vi "Force control.vi"() -> ()   [LabVIEW 2021]
uses:
  <vilib>/Platform/TimedLoop/XDataNode/timing_clust.ctl
  <vilib>/Platform/TimedLoop/XDataNode/nitl_modes.ctl
  <vilib>/Platform/TimedLoop/XDataNode/wakeup.ctl
  <vilib>/DAQmx/write.llb/DAQmx Write (Digital Bool 1Line 1Point).vi
  <vilib>/DAQmx/write.llb/DAQmx Write (Analog DBL 1Chan 1Samp).vi
  <vilib>/DAQmx/create/channels.llb/DAQmx Create Channel (AI-Voltage-Basic).vi
  <vilib>/DAQmx/create/channels.llb/DAQmx Create Channel (DO-Digital Output).vi
  <vilib>/DAQmx/create/channels.llb/DAQmx Create Channel (AO-Voltage-Basic).vi
  <vilib>/DAQmx/miscellaneous.llb/DAQmx Fill In Error Info.vi
  <vilib>/addons/control/pid/pid.llb/PID (DBL).vi
  <vilib>/Platform/TimedLoop/XDataNode/XDataNode.xnode
  <vilib>/Platform/TimedLoop/XDataNode/XDNodeRunTimeDep.lvlib
  <vilib>/addons/control/pid/NI_PID_pid.lvlib
panel:
  out "ff_gain 2":dbl
  in  "ff_gain":dbl(slide) scale=0.0..3.0
  out "predict":dbl
  out "Waveform Chart":cluster{"Filtered x":dbl, "Ref Force":dbl}(graph) caption="A"
  out "Total(V)":dbl
  in  "PID ON/OFF":bool
  in  "PID gains":T1={"proportional gain (Kc)"=0.3, "integral time (Ti, min)"=0.1, "derivative time (Td, min)"=0.0} {"derivative time (Td, min)" format="%.3f"; "integral time (Ti, min)" format="%.3f"; "proportional gain (Kc)" format="%.3f"}
  in  "Ref Force":dbl(slide) scale=0.0..40.0
  in  "Motor Enable":bool
  in  "stop":bool
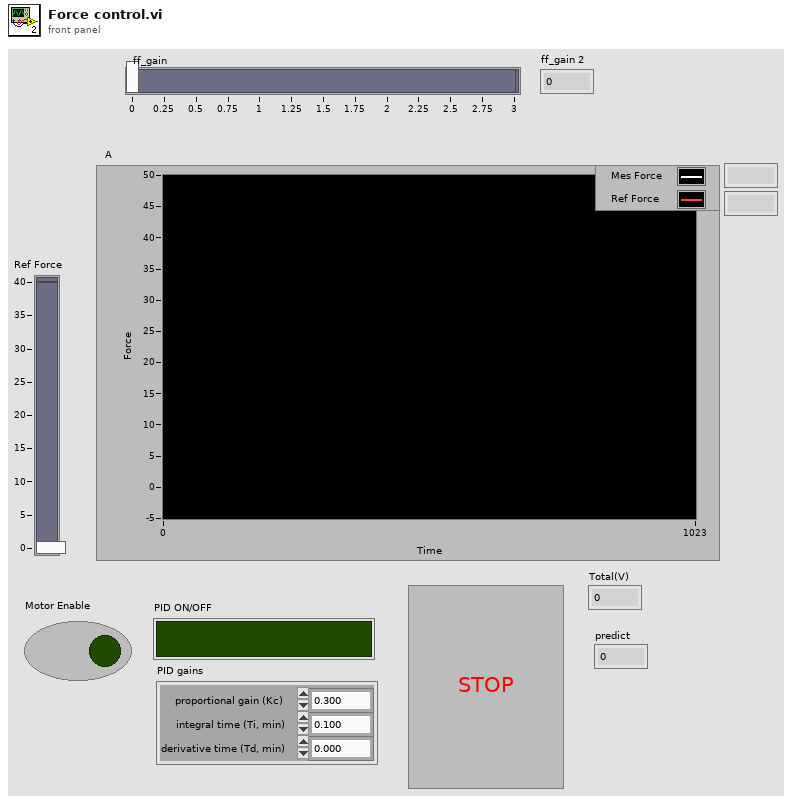
[diagram p1: front panel]
types:
  T1 = cluster{"proportional gain (Kc)":dbl, "integral time (Ti, min)":dbl, "derivative time (Td, min)":dbl}
  T2 = typedef "XDNodeRunTimeDep.lvlib/timing_clust.ctl" = cluster{"Expected End [f-1]":u64, "Actual End [f-1]":u64, "Finished Late? [f-1]":bool, "Expected End [i-1]":u64, "Actual End [i-1]":u64, "Finished Late? [i-1]":bool, "Expected Start [i]":u64, "Actual Start [i]":u64, "Expected Start [f]":u64, "Actual Start [f]":u64, "Source Name":string, "Structure Name":string, "Period":i64, "Deadline":i64, "Offset":i64, "Start":i64, "Priority":i32, "Timeout":i32, "Mode":T3, "Wakeup Reason":T4, "Error":errorcluster, "Source Type":string, "Secondary Source Type":string, "Global End Time":u64, "Global Start Time":u64, "Frame Duration":u64, "Iteration Duration":u64, "Assigned CPU":i32, "I/O Scan Engine Mode":u32}
  T3 = typedef "XDNodeRunTimeDep.lvlib/nitl_modes.ctl" = enum32{"No Change", "Process missed periods, maintain original phase", "Discard missed periods, maintain original phase", "Process missed periods, ignore original phase", "Discard missed periods, ignore original phase"}
  T4 = typedef "XDNodeRunTimeDep.lvlib/wakeup.ctl" = enum32{"Normal", "Aborted", "Asynchronous wakeup", "Timing source error", "Timed loop error", "Timeout"}
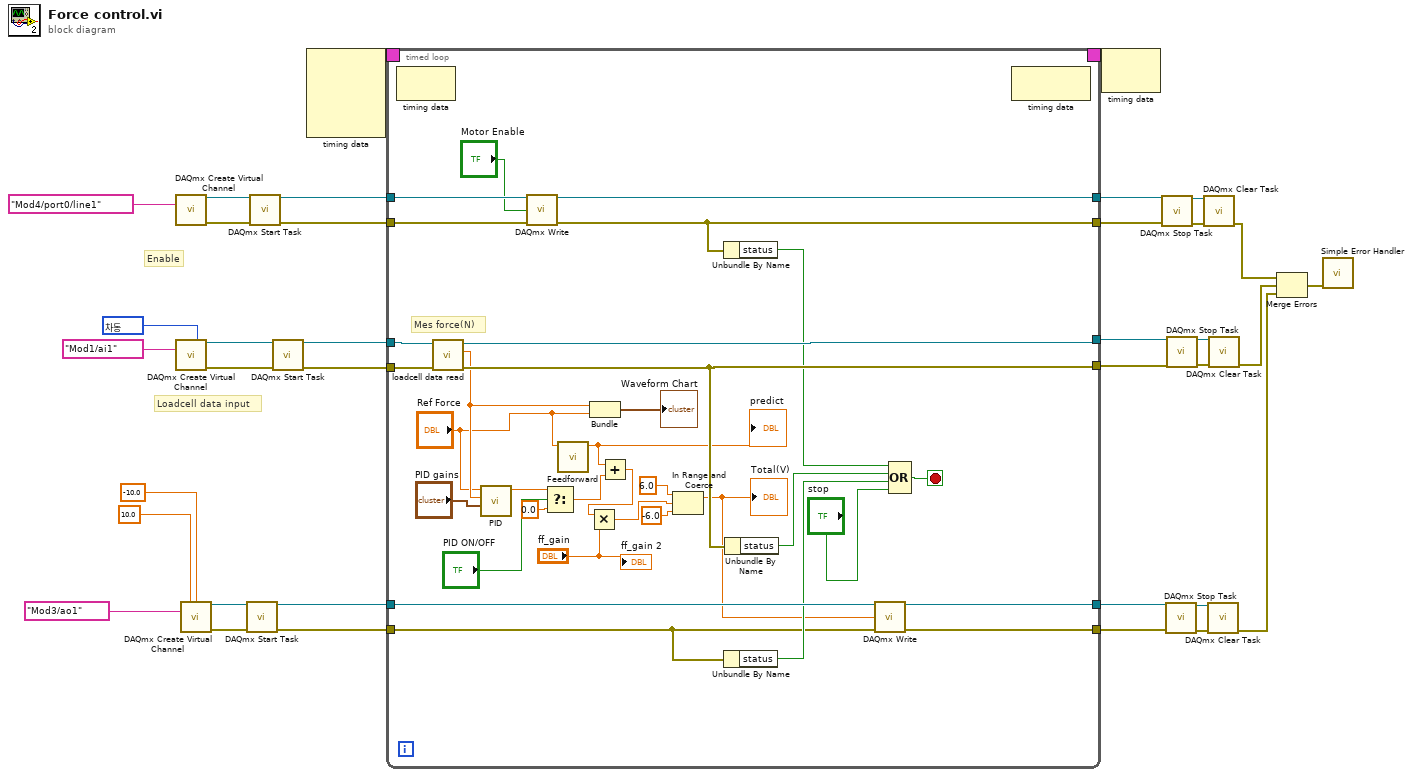
[diagram p0: block diagram]
diagram:
  w25 = 10106 items=["기본"=-1, "RSE"=10083, "NRSE"=10078, "차동"=10106, "유사 차동"=12529] ("input terminal configuration")
  # "Enable"
  # "Loadcell data input"
  n1 = call-poly <vilib>:"DAQmx Create Virtual Channel.vi"("lines"=tag "Mod4/port0/line1") -> ("task out"=w24:refnum<k21>, "error out"=w23:errorcluster)  [unwired: 13 in]
  n2 = call-poly <vilib>:"DAQmx Create Virtual Channel.vi"("input terminal configuration"=w25, "physical channels"=tag "Mod1/ai1") -> ("task out"=w33:refnum<k21>, "error out"=w32:errorcluster)  [unwired: 12 in]
  n3 = call-poly <vilib>:"DAQmx Create Virtual Channel.vi"("maximum value"=10.0, "minimum value"=-10.0, "physical channels"=tag "Mod3/ao1") -> ("task out"=w12:refnum<k21>, "error out"=w11:errorcluster)  [unwired: 11 in]
  n4 = call <vilib>:"DAQmx Start Task.vi"("task/channels in"=w12, "error in"=w11) -> ("task out"=w7:refnum<k21>, "error out"=w6:errorcluster)  [unwired: 12 in]
  n5 = call <vilib>:"DAQmx Start Task.vi"("task/channels in"=w24, "error in"=w23) -> ("task out"=w21:refnum<k21>, "error out"=w20:errorcluster)  [unwired: 12 in]
  n6 = call <vilib>:"DAQmx Start Task.vi"("task/channels in"=w33, "error in"=w32) -> ("task out"=w31:refnum<k21>, "error out"=w30:errorcluster)  [unwired: 12 in]
  n7 = node-c288() -> (w36:T2)  [unwired: 4 in]
  n8 = timed-loop {
    timing: w36 -> [_]
    timing-out: [_] -> w35
    tunnel: w31 -> [w69]
    tunnel: w30 -> [w68]
    tunnel: [w67] -> w26
    tunnel: [w66] -> w27
    tunnel: w21 -> [w63]
    tunnel: w20 -> [w62]
    tunnel: [w60] -> w17
    tunnel: [w59] -> w16
    tunnel: w7 -> [w57]
    tunnel: w6 -> [w52]
    tunnel: [w56] -> w3
    tunnel: [w55] -> w2
    stop <- w64 stop-if-true
    # "Mes force(N)"
    n9 = node-c288() -> ()  [unwired: 1 in, 1 out]
    n10 = call "loadcell data read.vi"("error in (no error)"=w68, "Refnum in"=w69) -> ("error out"=w66:errorcluster, "Filtered x"=w44:dbl, "Refnum out"=w67:refnum<k21>)  [unwired: 7 in]
    n11 = call-poly <vilib>:"PID.vi"("PID gains"="PID gains", "process variable"=w44, "setpoint"="Ref Force") -> ("output"=w50:dbl)  [unwired: 7 in, 1 out]
    n12 = call-poly <vilib>:"DAQmx Write.vi"("task/channels in"=w63, "data"="Motor Enable", "error in"=w62) -> ("task out"=w60:refnum<k21>, "error out"=w59:errorcluster)  [unwired: 10 in, 1 out]
    n13 = Select(t=w50, s="PID ON/OFF", f=0.0) -> (s? t:f=w40:dbl)
    n14 = call "Feedforward.vi"("Ref force"="Ref Force") -> ("predict"=w41:dbl)  [unwired: 10 in]
    "predict" <- w41
    n15 = Bundle("Filtered x"=w44, "Ref Force"="Ref Force") -> (→"Waveform Chart":cluster{"Filtered x":dbl, "Ref Force":dbl})  [unwired: 1 in]
    n16 = Add(x=w41, y=w40) -> (x+y=w39:dbl)
    n17 = Multiply(x=w39, y="ff_gain") -> (x*y=w38:dbl)
    n18 = In Range and Coerce(upper limit=6.0, x=w38, lower limit=-6.0) -> (coerced(x)=w45:dbl)  [unwired: 1 out]
    "Total(V)" <- w45
    n19 = Unbundle By Name(w59) -> ("status"=w58:bool)
    n20 = Unbundle By Name(w52) -> ("status"=w54:bool)
    n21 = Unbundle By Name(w66) -> ("status"=w65:bool)
    n22 = call-poly <vilib>:"DAQmx Write.vi"("task/channels in"=w57, "data"=w45, "error in"=w52) -> ("task out"=w56:refnum<k21>, "error out"=w55:errorcluster)  [unwired: 10 in, 1 out]
    n23 = Compound Arithmetic op=OR(w58, w65, w54, "stop") -> (w64:bool)
    n24 = node-c288() -> ()  [unwired: 1 in, 1 out]
    "ff_gain 2" <- "ff_gain"
  }
  n25 = node-c288(w35) -> ()  [unwired: 1 out]
  n26 = call <vilib>:"DAQmx Stop Task.vi"("task/channels in"=w17, "error in"=w16) -> ("task out"=w19:refnum<k21>, "error out"=w18:errorcluster)  [unwired: 12 in]
  n27 = call <vilib>:"DAQmx Stop Task.vi"("task/channels in"=w3, "error in"=w2) -> ("task out"=w5:refnum<k21>, "error out"=w4:errorcluster)  [unwired: 12 in]
  n28 = call <vilib>:"DAQmx Stop Task.vi"("task/channels in"=w26, "error in"=w27) -> ("task out"=w29:refnum<k21>, "error out"=w28:errorcluster)  [unwired: 12 in]
  n29 = call <vilib>:"DAQmx Clear Task.vi"("task in"=w19, "error in"=w18) -> ("error out"=w15:errorcluster)  [unwired: 13 in]
  n30 = call <vilib>:"DAQmx Clear Task.vi"("task in"=w5, "error in"=w4) -> ("error out"=w1:errorcluster)  [unwired: 13 in]
  n31 = call <vilib>:"DAQmx Clear Task.vi"("task in"=w29, "error in"=w28) -> ("error out"=w14:errorcluster)  [unwired: 13 in]
  n32 = Merge Errors(w15, w14, w1) -> (w13:errorcluster)
  n33 = call <vilib>:"Simple Error Handler.vi"("error in (no error)"=w13) -> ()  [unwired: 4 in, 5 out]
